vi "Definition Cluster.vi"(11 "Entity Collection in":refnum<class "Entity Collection.lvclass">) -> (2 "Definition":variant, 3 "Entity Collection out":refnum<class "Entity Collection.lvclass">)   [LabVIEW 2020, in "Conditu2.lvlib" / "Columns.lvlib" / "Entity Collection.lvclass"]
uses:
  Entity Collection.lvclass
  C:/dev/lv20CE/lv-conditum-tools/Conditum-Clone/Columns/Relation/Relation.lvclass
  Collection Definition.ctl
  Relation/Relation Info.ctl
  Relation Mapping.ctl
  Conditu2.lvlib
  Relation/Relation.lvclass
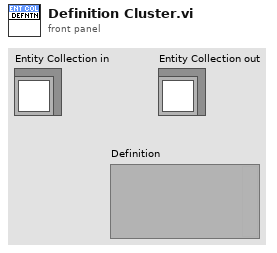
[diagram p1: front panel]
types:
  T1 = typedef "Conditu2.lvlib/Columns.lvlib/Entity Collection.lvclass/Collection Definition.ctl" = cluster{"Table Name":string, "Relation":T2}
  T2 = typedef "Conditu2.lvlib/Relation Info.ctl" = cluster{"Mapping":T3, "Related To":string, "Reversed By":string}
  T3 = typedef "Conditu2.lvlib/Relation Mapping.ctl" = enum16{"OneToOne", "OneToMany", "ManyToOne", "ManyToMany"}
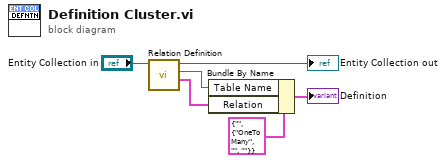
[diagram p0: block diagram]
diagram:
  n1 = call "Relation Definition.vi"("Relation in"="Entity Collection in") -> ("Relation Definition"=w1:T2, "Table Name"=w2:string, "Relation out"=→"Entity Collection out":refnum<class "Entity Collection.lvclass">)  [unwired: 8 in]
  n2 = Bundle By Name(cluster=T1 {"Table Name"="", "Relation"={"Mapping"=enum."OneToMany", "Related To"="", "Reversed By"=""}} ("Collection Definition"), "Table Name"=w2, "Relation"=w1) -> (→"Definition":T1)
